vi "I2Csetpixels.vi"(0 "I2C Reference In":string, 1 "Color Box":u32, 5 "Brightness (0-255)":u8, 7 "RGB Array":u8[](array[numeric]), 9 "LED Position":u8, 11 "Error In":errorcluster, 12 "InputSelect":enum16{"RGB", "ColorBox"}(ring)) -> (3 "Resolved Color":u32 format="%.0x", 4 "I2C Reference Out":T1 {"Device Address" format="%.0x"}, 6 "R":u8, 8 "G":u8, 10 "B":u8, 15 "Error Out":errorcluster)   [LabVIEW 2014]
uses:
  <vilib>/Rock Robotics/WPI/I2C/WPI_I2CDevRef.ctl
  <vilib>/Rock Robotics/SystemInterfaces/Typedef/FPGA_TypedefDigitalModule.ctl
  <vilib>/Rock Robotics/SystemInterfaces/i2clib/i2c_bus.ctl
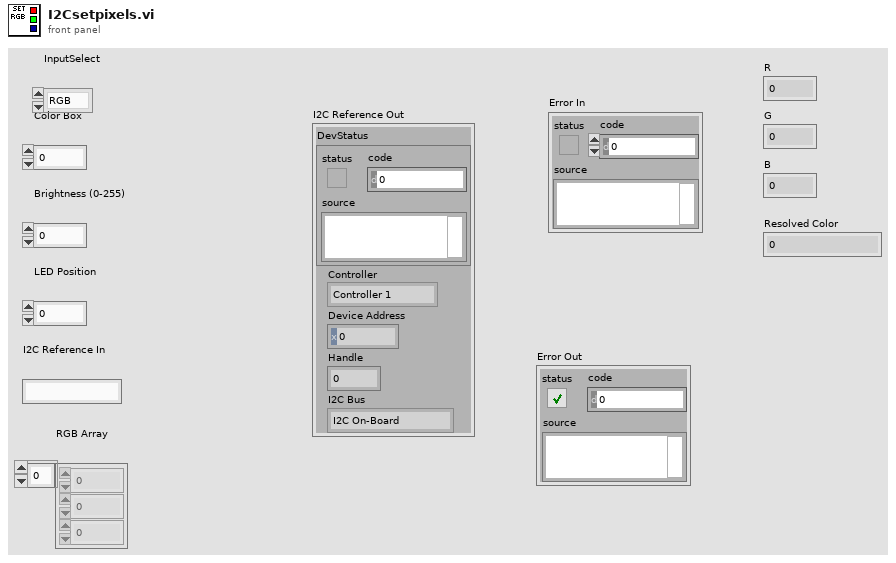
[diagram p1: front panel]
types:
  T1 = typedef "WPI_I2CDevRef.ctl" = cluster{"DevStatus":errorcluster, "Controller":T2, "Device Address":u8, "Handle":i32, "I2C Bus":T3}
  T2 = typedef "FPGA_TypedefDigitalModule.ctl" = enum16{"Controller 1"}
  T3 = typedef "i2c_bus.ctl" = enum16{"I2C On-Board", "I2C MXP", "Invalid"}
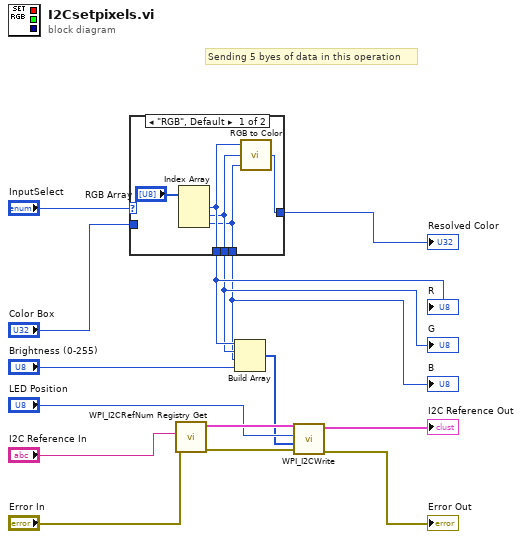
[diagram p0: block diagram]
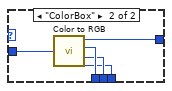
[diagram p2: hidden frame]
diagram:
  # "Sending 5 byes of data in this operation"
  n1 = case shown="\"RGB\", Default" "InputSelect" {
    tunnel: [w19 w25] -> w10
    tunnel: "Color Box" -> [_ w24]
    tunnel: [w16 w23] -> w4
    tunnel: [w18 w22] -> w3
    tunnel: [w17 w21] -> w2
    frame "RGB", Default {
      n2 = Index Array(array="RGB Array") -> (element #1=w19:u8, element #2=w18:u8, element #3=w17:u8)  [unwired: 3 in]
      n3 = call <vilib>:"RGB to Color.vi"("B"=w17, "G"=w18, "R"=w19) -> ("Color"=w16:u32)
    }
    frame "ColorBox" {
      n4 = call <vilib>:"Color to RGB.vi"("Color"=w24) -> ("Resolved Color"=w23:u32, "R"=w25:u8, "G"=w22:u8, "B"=w21:u8)
    }
  }
  "Resolved Color" <- w4
  "R" <- w10
  "G" <- w3
  "B" <- w2
  n5 = call <vilib>:"WPI_I2CRefNum Registry Get.vi"("error in (no error)"="Error In", "refnum name"="I2C Reference In") -> ("error out"=w15:errorcluster, "I2CDevRef"=w14:T1)  [unwired: 8 in]
  n6 = Build Array(w10, w3, w2, "Brightness (0-255)") -> (w11:u8[])
  n7 = call <vilib>:"WPI_I2CWrite.vi"("error in (no error)"=w15, "I2CDataToSend"=w11, "I2CRegister"="LED Position", "I2CDevRef"=w14) -> ("error out"=→"Error Out":errorcluster, "I2CDevRef"=→"I2C Reference Out":T1)  [unwired: 6 in]
